vi "Create ListView Ref.vi"(8 "error in (no error)":errorcluster caption="错误输入（无错误）", 11 "ListView":refnum<k24>) -> (0 "error out":errorcluster caption="错误输出", 3 "ListViewClass 输出":refnum<class "ListViewClass.lvclass"> caption="DNL_LabVIEW Object out")   [LabVIEW 2012, in "ListViewClass.lvclass"]
uses:
  ListViewClass.lvclass
  System.Windows.Forms
  ListViewClass.lvclass/ListViewClass.ctl
panel:
  in  "ListViewClass 输入":refnum<class "ListViewClass.lvclass"> caption="DNL_LabVIEW Object in"
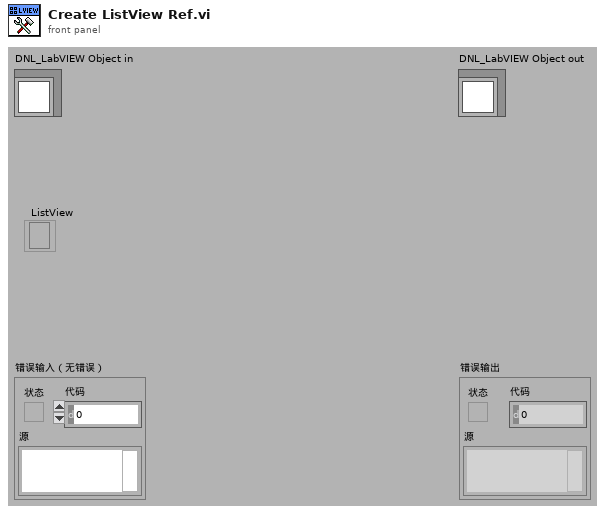
[diagram p1: front panel]
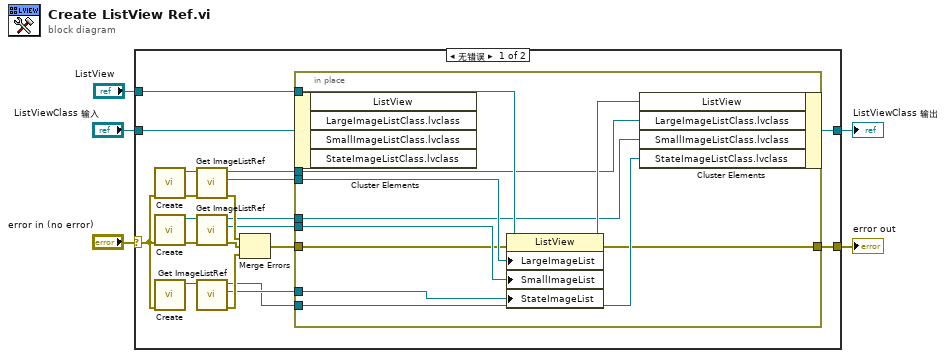
[diagram p0: block diagram]
diagram:
  n1 = case shown="无错误" "error in (no error)" {
    selector: "error in (no error)" -> [w17 w37]
    tunnel: [w7 w37] -> w4
    tunnel: [w24 w36] -> w2
    tunnel: "ListViewClass 输入" -> [w25 w36]
    tunnel: "ListView" -> [w23 _]
    frame No Error {
      n2 = call "Create.vi"("error in (no error)"=w17) -> ("error out"=w21:errorcluster, "ImageListClass 输出"=w18:refnum<class "ImageListClass.lvclass">)  [unwired: 9 in]
      n3 = call "Create.vi"("error in (no error)"=w17) -> ("error out"=w22:errorcluster, "ImageListClass 输出"=w19:refnum<class "ImageListClass.lvclass">)  [unwired: 9 in]
      n4 = call "Create.vi"("error in (no error)"=w17) -> ("ImageListClass 输出"=w20:refnum<class "ImageListClass.lvclass">)  [unwired: 9 in, 1 out]
      n5 = call "Get ImageListRef.vi"("error in (no error)"=w21, "ImageListClass 输入"=w18) -> ("error out"=w16:errorcluster, "ImageList"=w13:refnum<k24>, "ImageListClass 输出"=w10:refnum<class "ImageListClass.lvclass">)  [unwired: 7 in]
      n6 = call "Get ImageListRef.vi"("error in (no error)"=w22, "ImageListClass 输入"=w19) -> ("error out"=w15:errorcluster, "ImageList"=w12:refnum<k24>, "ImageListClass 输出"=w9:refnum<class "ImageListClass.lvclass">)  [unwired: 7 in]
      n7 = call "Get ImageListRef.vi"("ImageListClass 输入"=w20) -> ("error out"=w14:errorcluster, "ImageList"=w11:refnum<k24>, "ImageListClass 输出"=w8:refnum<class "ImageListClass.lvclass">)  [unwired: 8 in]
      n8 = Merge Errors(w16, w15, w14) -> (w6:errorcluster)
      n9 = in-place {
        in-place-border: w23 -> [w34]
        in-place-border: w13 -> [w33]
        in-place-border: w12 -> [w32]
        in-place-border: w11 -> [w31]
        in-place-border: w10 -> [w30]
        in-place-border: w9 -> [w29]
        in-place-border: w8 -> [w28]
        in-place-border: [w27] -> w7
        in-place-border: w6 -> [w26]
        n10 = in-place-cluster #1(w25) -> ()  [unwired: 4 out]
        n11 = property class="ListView"(reference=w34, error in=w26, "LargeImageList"=w33, "SmallImageList"=w32, "StateImageList"=w31) -> (reference out=w35:refnum<k24>, error out=w27:errorcluster)
        n12 = in-place-cluster #1("ListView"=w35, "LargeImageListClass.lvclass"=w30, "SmallImageListClass.lvclass"=w29, "StateImageListClass.lvclass"=w28) -> (w24:refnum<class "ListViewClass.lvclass">)
      }
    }
    frame Error {
    }
  }
  "error out" <- w4
  "ListViewClass 输出" <- w2
